vi "Client.vi"() -> ()   [LabVIEW 2020]
panel:
  out "Chart":dbl(graph)
  in  "Enum":enum16{"Acq1", "Acq2", ""}(ring)
  in  "stop":bool
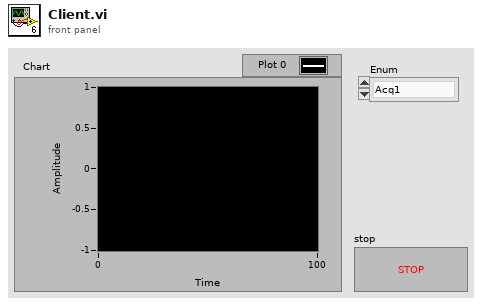
[diagram p1: front panel]
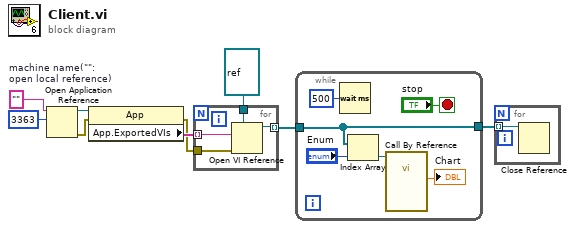
[diagram p0: block diagram]
diagram:
  w2 = ""  # machine name("":  open local reference)
  n1 = Open Application Reference(10:u16 3363 ("port number or service name (3363)"), 11:w2) -> (0:w8:errorcluster, 3:w9:refnum<vi>)  [unwired: 2 in]
  n2 = property class="App"(reference=w9, error in=w8) -> (error out=w6:errorcluster, "App.ExportedVIs"=w7:string[])  [unwired: 1 out]
  n3 = for {
    tunnel: w7 -> [w13] mode=indexing
    tunnel: w6 -> [w12]
    tunnel: [w11] -> w5 mode=indexing
    tunnel: refnum<vi> refnum ("type specifier VI Refnum (for type only)") -> [w10]
    n4 = Open VI Reference(type specifier VI Refnum (for type only)=w10, vi path=w13, error in (no error)=w12) -> (vi reference=w11:refnum<vi>)  [unwired: 3 in, 1 out]
  }
  n5 = while {
    tunnel: w5 -> [w16]
    tunnel: [w16] -> w3
    stop <- "stop" stop-if-true
    n6 = Wait (ms)(milliseconds to wait=u32 500) -> ()  [unwired: 1 out]
    n7 = Index Array(array=w16, index="Enum") -> (element=w15:refnum<vi>)
    n8 = call-by-ref "?"(reference=w15) -> ("sin(x)"=→"Chart":dbl)  [unwired: 12 in, 2 out]
  }
  n9 = for {
    tunnel: w3 -> [w20] mode=indexing
    n10 = Close Reference(reference=w20) -> ()  [unwired: 1 in, 1 out]
  }
